vi "only_trigger.vi"() -> ()   [LabVIEW 2019]
uses:
  <vilib>/Platform/TimedLoop/XDataNode/timing_clust.ctl
  <vilib>/Platform/TimedLoop/XDataNode/nitl_modes.ctl
  <vilib>/Platform/TimedLoop/XDataNode/wakeup.ctl
  <vilib>/FPGAPlugInAG/myRIO-1900/niLvFpga_Open_myRIO-1900.vi
  <vilib>/rvi/interface/common/dynamic/niFpgaDynamicAddResources.vi
  <vilib>/Utility/error.llb/Error Cluster From Error Code.vi
  <vilib>/rvi/errors/niLvFpgaAdjustHostInterfaceError.vi
  <vilib>/FPGAPlugInAG/Dynamic/niLvFpga_Close_Dynamic.vi
  <vilib>/Platform/TimedLoop/XDataNode/XDataNode.xnode
  <vilib>/rvi/interface/nirviOpenFPGA/nirviOpenFPGA.xnode
  FPGA Bitfiles/capstone_FPGATarget_encoderFPGA_AeXAVEDpCcY.lvbitx
  encoder_FPGA.vi
  <vilib>/rvi/interface/nirviReadWriteControl/nirviReadWriteControl.xnode
  <vilib>/rvi/interface/nirviCloseFPGA/nirviCloseFPGA.xnode
  <vilib>/Platform/TimedLoop/XDataNode/XDNodeRunTimeDep.lvlib
  NiFpgaLv.dll
  <vilib>/rvi/interface/Simulation/niFpgaSimulationCallBeginRW.vi
panel:
  out "숫자형":i32
  in  "tir_Enable (escon)":bool
  in  "뒷 정지":bool
  in  "stop":bool
  in  "pwm input(escon)":i32
  out "Timeout":i32
  out "Encoder  (4x)":i32
  in  "DIR":bool
  out "현재상태":string
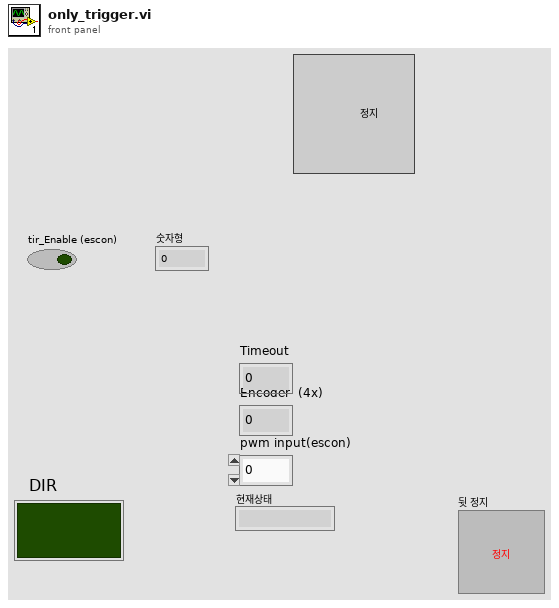
[diagram p1: front panel]
types:
  T1 = typedef "XDNodeRunTimeDep.lvlib/timing_clust.ctl" = cluster{"Expected End [f-1]":u64, "Actual End [f-1]":u64, "Finished Late? [f-1]":bool, "Expected End [i-1]":u64, "Actual End [i-1]":u64, "Finished Late? [i-1]":bool, "Expected Start [i]":u64, "Actual Start [i]":u64, "Expected Start [f]":u64, "Actual Start [f]":u64, "Source Name":string, "Structure Name":string, "Period":i64, "Deadline":i64, "Offset":i64, "Start":i64, "Priority":i32, "Timeout":i32, "Mode":T2, "Wakeup Reason":T3, "Error":errorcluster, "Source Type":string, "Secondary Source Type":string, "Global End Time":u64, "Global Start Time":u64, "Frame Duration":u64, "Iteration Duration":u64, "Assigned CPU":i32, "I/O Scan Engine Mode":u32}
  T2 = typedef "XDNodeRunTimeDep.lvlib/nitl_modes.ctl" = enum32{"No Change", "Process missed periods, maintain original phase", "Discard missed periods, maintain original phase", "Process missed periods, ignore original phase", "Discard missed periods, ignore original phase"}
  T3 = typedef "XDNodeRunTimeDep.lvlib/wakeup.ctl" = enum32{"Normal", "Aborted", "Asynchronous wakeup", "Timing source error", "Timed loop error", "Timeout"}
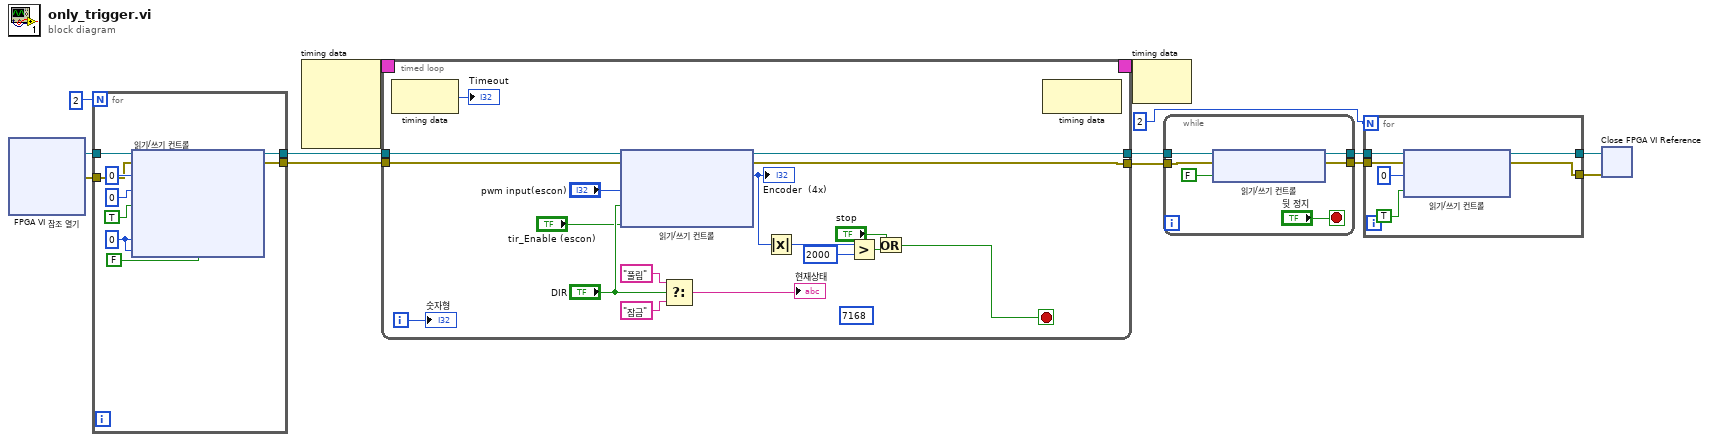
[diagram p0: block diagram]
diagram:
  n1 = xnode "FPGA VI 참조 열기"() -> ("FPGA VI 참조 출력"=w4:refnum<k20>, "에러 출력"=w3:errorcluster)  [unwired: 2 in]
  n2 = for {
    N: 2 -> [_]
    tunnel: [w23] -> w12
    tunnel: [w22] -> w11
    tunnel: w4 -> [w16]
    tunnel: w3 -> [w15]
    w17 = 0 ("직동_pwm input")
    n3 = xnode "읽기/쓰기 컨트롤"("FPGA VI 참조 입력"=w16, "에러 입력"=w15, "tir_Encoder  (4x)"=0 ("Encoder  (4x)"), "tir_pwm input(escon)"=0 ("pwm input(escon)"), "tir_encoder reset"=TRUE ("encoder reset"), "직동_pwm input"=w17, "tir_Enable (escon)"=FALSE, "pwm input"=w17) -> ("FPGA VI 참조 출력"=w23:refnum<k20>, "에러 출력"=w22:errorcluster)
  }
  n4 = node-c288() -> (w14:T1)  [unwired: 4 in]
  n5 = timed-loop {
    timing: w14 -> [_]
    timing-out: [_] -> w13
    tunnel: w12 -> [w41]
    tunnel: w11 -> [w40]
    tunnel: [w25] -> w2
    tunnel: [w24] -> w1
    i -> [w26]
    stop <- w30 stop-if-true
    (unwired) 7168 ("y")
    n6 = node-c288() -> (→"Timeout":i32)  [unwired: 1 in]
    n7 = xnode "읽기/쓰기 컨트롤"("FPGA VI 참조 입력"=w41, "에러 입력"=w40, "tir_pwm input(escon)"="pwm input(escon)", "tir_DIR"="DIR", "tir_Enable (escon)"="tir_Enable (escon)") -> ("FPGA VI 참조 출력"=w25:refnum<k20>, "에러 출력"=w24:errorcluster, "tir_Encoder  (4x)"=w33:i32)
    "Encoder  (4x)" <- w33
    n8 = Select(t="풀림", s="DIR", f="잠금") -> (s? t:f=→"현재상태":string)
    n9 = Absolute Value(x=w33) -> (abs(x)=w32:i32)
    n10 = Greater?(x=w32, y=2000) -> (0:w37:bool)
    n11 = Or(x="stop", y=w37) -> (x .or. y?=w30:bool)
    n12 = node-c288() -> ()  [unwired: 1 in, 1 out]
    "숫자형" <- w26
  }
  n13 = node-c288(w13) -> ()  [unwired: 1 out]
  n14 = while {
    tunnel: [w50] -> w9
    tunnel: [w49] -> w8
    tunnel: w2 -> [w46]
    tunnel: w1 -> [w45]
    stop <- "뒷 정지" stop-if-true
    n15 = xnode "읽기/쓰기 컨트롤"("FPGA VI 참조 입력"=w46, "에러 입력"=w45, "tir_Enable (escon)"=FALSE ("Enable (escon)")) -> ("FPGA VI 참조 출력"=w50:refnum<k20>, "에러 출력"=w49:errorcluster)
  }
  n16 = for {
    N: 2 -> [_]
    tunnel: w9 -> [w56]
    tunnel: w8 -> [w54]
    tunnel: [w52] -> w6
    tunnel: [w51] -> w5
    n17 = xnode "읽기/쓰기 컨트롤"("FPGA VI 참조 입력"=w56, "에러 입력"=w54, "tir_Encoder  (4x)"=0 ("Encoder  (4x)"), "tir_encoder reset"=TRUE ("Enable (escon)")) -> ("FPGA VI 참조 출력"=w52:refnum<k20>, "에러 출력"=w51:errorcluster)
  }
  n18 = xnode "Close FPGA VI Reference"("FPGA VI 참조 입력"=w6, "에러 입력"=w5) -> ()  [unwired: 1 out]
